vi "Get Unique Test ID.vi"(1 "GPIB Board in":refnum<class "GPIB Board Design.lvclass">) -> (0 "ID #":u32)   [LabVIEW 2023, in "GPIB Board Design.lvclass"]
doc: "Get an identification number."
uses:
  GPIB Board Design.lvclass
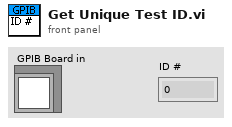
[diagram p1: front panel]
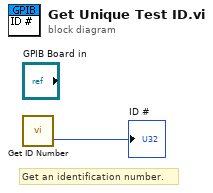
[diagram p0: block diagram]
diagram:
  # "Get an identification number."
  n1 = call "Get ID Number.vi"() -> ("id number"=→"ID #":u32)  [unwired: 2 in]
